vi "EnableVisionLogic (SubVI).vi"(9 "Activate?(hold)":bool, 10 "Offset(degrees)":dbl, 11 "Target?":bool) -> (3 "Enable?":bool)   [LabVIEW 2018]
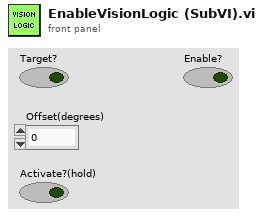
[diagram p1: front panel]
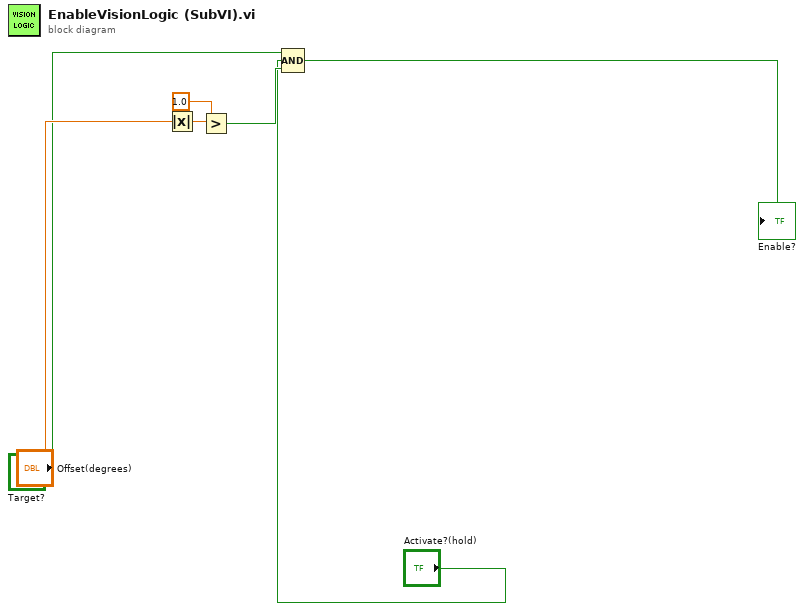
[diagram p0: block diagram]
diagram:
  n1 = Absolute Value(x="Offset(degrees)") -> (abs(x)=w4:dbl)
  n2 = Greater?(x=w4, y=1.0) -> (0:w5:bool)
  n3 = Compound Arithmetic op=AND("Target?", "Activate?(hold)", w5) -> (→"Enable?":bool)
